vi "_Main.vi"(10 "Camera Occurance":refnum<k4>) -> ()   [LabVIEW 2017, in "VisionHW.lvlib"]
uses:
  VisionHW.lvlib
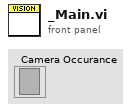
[diagram p1: front panel]
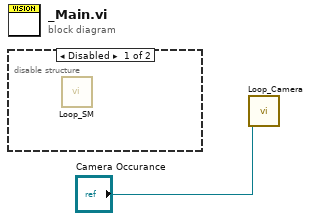
[diagram p0: block diagram]
diagram:
  n1 = disable-structure shown="Disabled" {
    frame Disabled {
      n2 = call "Loop_SM.vi"() -> ()  [unwired: 12 in]
    }
    frame Enabled {
    }
  }
  n3 = call "Loop_Camera.vi"("Camera Occurance"="Camera Occurance") -> ()  [unwired: 11 in]
